vi "lab7_Avoid obstacle button2.0 - kpfinal.vi"() -> ()   [LabVIEW 2018]
uses:
  <userlib>/KNR OS 3.0 LabVIEW Toolkit/Type Definition/Resource.ctl
  <userlib>/KNR OS 3.0 LabVIEW Toolkit/Type Definition/DC Motor Port.ctl
  <userlib>/KNR OS 3.0 LabVIEW Toolkit/Type Definition/Ultrasonic Port Number.ctl
  <vilib>/myRIO/Common/Instrument Driver Framework/myRIO v1.0/UART/vis/myRIO v1.0 Close UART.vi
  <vilib>/myRIO/Common/Instrument Driver Framework/Utilities/vis/FPGA Ref Manager.vi
  <vilib>/myRIO/Common/Instrument Driver Framework/myRIO v1.0/myRIO v1.0 Reset FPGA.vi
  <vilib>/myRIO/Common/Instrument Driver Framework/myRIO v1.0/IRQ/vis/myRIO v1.0 IRQ Info FGV.vi
  <vilib>/myRIO/Common/Instrument Driver Framework/myRIO v1.0/IRQ/vis/myRIO v1.0 Timer IRQ Info FGV.vi
  <vilib>/myRIO/Common/Instrument Driver Framework/myRIO v1.0/IRQ/vis/myRIO v1.0 ISR Agent.vi
  <vilib>/myRIO/Instrument Drivers/Utilities/Utilities.lvlib
panel:
  out "Velocity R (cm/s)":dbl=3750.0
  out "Velocity L":dbl=-2062.5
  in  "stop":bool
  in  "kp":dbl=5.8 format="%#_13g"
  out "Speed R 2":dbl=4.06
  out "Speed L 2":dbl=4.06
  in  "upper limit R":dbl=15.0
  in  "upper limit L":dbl=20.0
  in  "Speed":dbl=8.0
  in  "Distance":dbl=35.0
  in  "Kp":dbl=0.3
  in  "Reverse Encoder R":bool=TRUE
  in  "Reverse Encoder L":bool=TRUE
  in  "Y":dbl=-5.0
  in  "X":dbl=190.0
  out "Pos R":dbl=170.41358455446547
  out "Pos L":dbl=162.57741982327175
  out "Actual X":dbl=165.0804505801855
  out "Actual Y":dbl=-0.734330747670838
  out "Theta":dbl=21.37996031746032 caption="Heading"
  in  "Reset Encoder R":bool
  in  "Reset Encoder L":bool
  in  "L set Us":dbl=45.0 format="%#_13g"
  in  "Mid set IR":dbl=46.0 format="%#_13g"
  in  "R set Us":dbl=25.0 format="%#_13g"
  out "Case":dbl
  out "L":dbl(slide)=299.99420158565044 scale=0.0..300.0
  out "mid":dbl(slide)=1010.0268999999998 scale=0.0..300.0
  out "R":dbl(slide)=262.09784746170044 scale=0.0..300.0
  out "L Us":dbl=299.99420158565044
  out "MID Us":dbl=1010.0268999999998
  out "R Us":dbl=262.09784746170044
  in  "?":bool
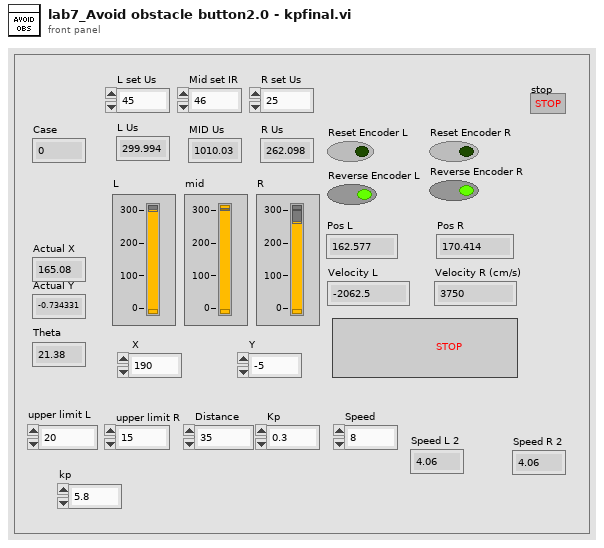
[diagram p1: front panel]
types:
  T1 = typedef "DC Motor Port.ctl" = u16
  T2 = typedef "Resource.ctl" = enum16{"KNRm_DDRC", "KNRm_DDDD", "KNRm_DDDR", "KNRm_DDDC", "KNR"}
  T3 = typedef "KNR3 Reference.ctl" = cluster{"FPGA Session":refnum<class "FPGA Interface Base.lvclass">, "Resource":T2}
  T4 = typedef "Ultrasonic Port Number.ctl" = u16
  T5 = cluster{"Dist 1(cm)":dbl, "Dist 2(cm)":dbl, "Dist 3 (cm)":dbl, "Dist 4 (cm)":dbl}
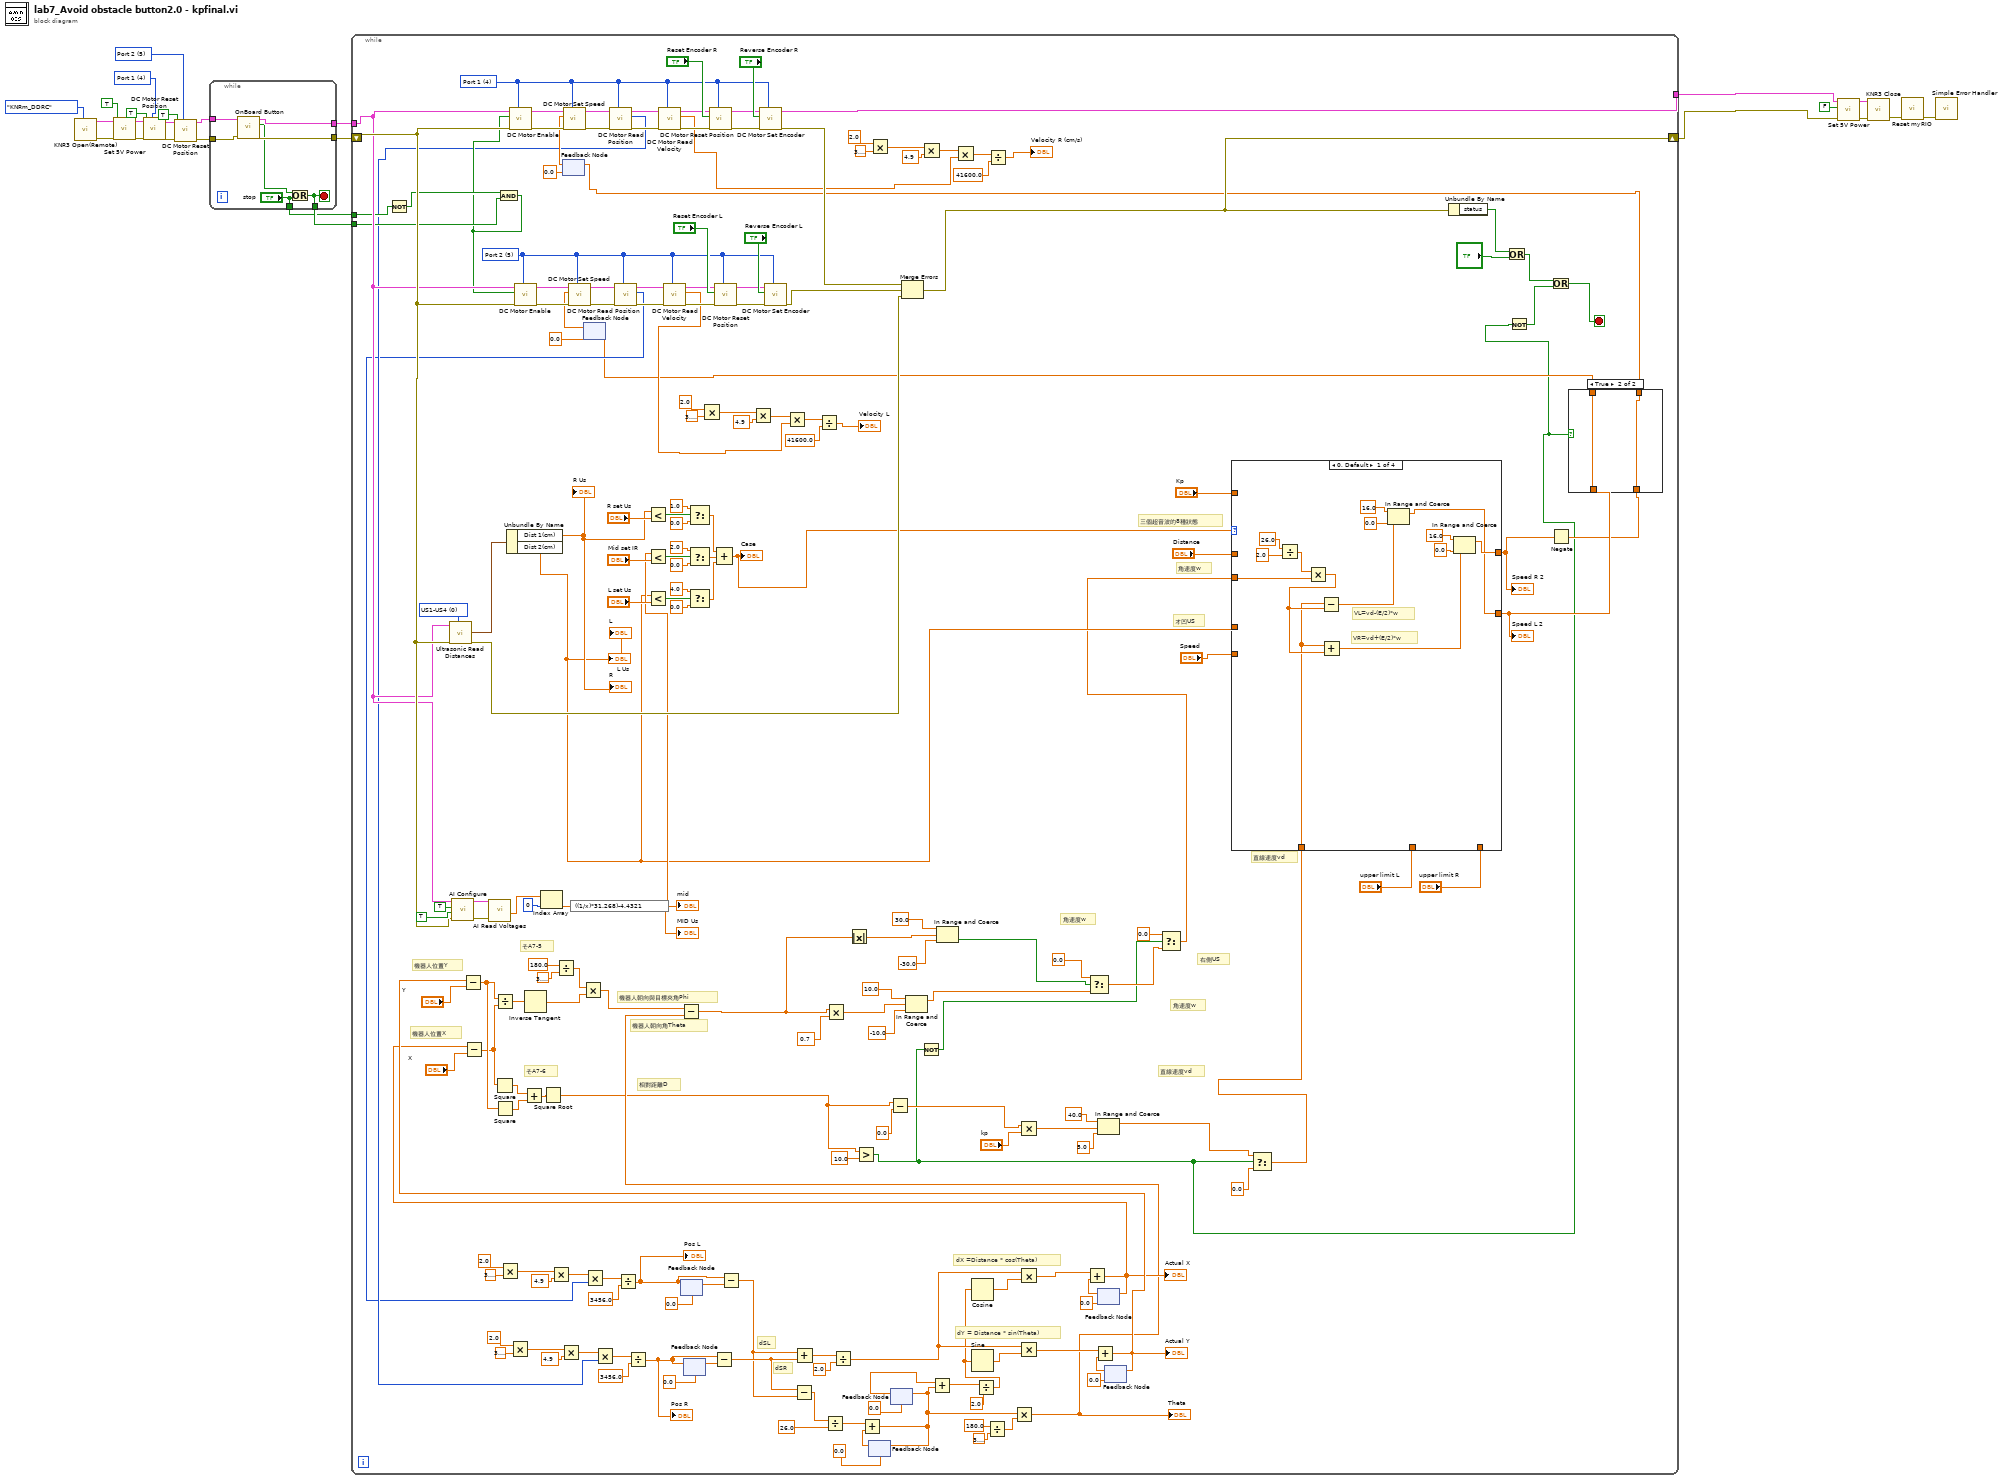
[diagram p0: block diagram]
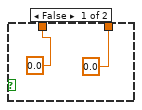
[diagram p2: hidden frame]
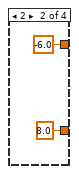
[diagram p3: hidden frame]
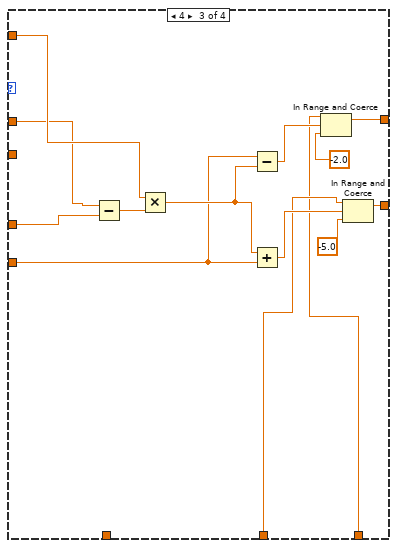
[diagram p4: hidden frame]
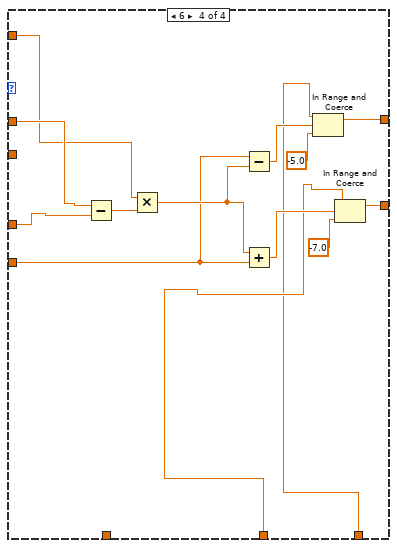
[diagram p5: hidden frame]
diagram:
  w11 = T1 5 items=["Port 1"=4, "Port 2"=5, "Port 3"=6, "Port 4"=7, "Port 5"=8, "Port 6"=9, "Port 7"=10] ("Port Number 2")
  w12 = T1 4 items=["Port 1"=4, "Port 2"=5, "Port 3"=6, "Port 4"=7, "Port 5"=8, "Port 6"=9, "Port 7"=10] ("Port Number")
  n1 = call <userlib>:"KNR3 Open(Remote).vi"("Resource"=Resource."KNRm_DDRC") -> ("error out"=w20:errorcluster, "KNR out"=w21:T3)  [unwired: 9 in]
  n2 = call <userlib>:"Set 5V Power.vi"("error in (no error)"=w20, "5V Power(T)"=TRUE ("5V Power"), "KNR in"=w21) -> ("error out"=w13:errorcluster, "KNR out"=w16:T3)  [unwired: 7 in]
  n3 = call <userlib>:"DC Motor Reset Position.vi"("Port (DS1)"=w12, "error in (no error)"=w13, "Reset(F)"=TRUE, "KNR in"=w16) -> ("error out"=w14:errorcluster, "KNR out"=w15:T3)  [unwired: 6 in]
  n4 = call <userlib>:"DC Motor Reset Position.vi"("Port (DS1)"=w11, "error in (no error)"=w14, "Reset(F)"=TRUE, "KNR in"=w15) -> ("error out"=w7:errorcluster, "KNR out"=w6:T3)  [unwired: 6 in]
  n5 = while {
    tunnel: [w32] -> w8
    tunnel: w7 -> [w31]
    tunnel: w6 -> [w30]
    tunnel: [w29] -> w5
    tunnel: [w27] -> w4
    tunnel: ["stop"] -> w3
    stop <- w27 stop-if-true
    n6 = call <userlib>:"OnBoard Button.vi"("error in (no error)"=w31, "KNR in"=w30) -> ("error out"=w32:errorcluster, "value"=w28:bool, "KNR out"=w29:T3)  [unwired: 7 in]
    n7 = Or(x=w28, y="stop") -> (x .or. y?=w27:bool)
  }
  n8 = while {
    tunnel: [w219] -> w2
    shift-right: [w205] -> w1
    shift-left: w8 -> [w168]
    tunnel: w5 -> [w91]
    tunnel: w4 -> [w90]
    tunnel: w3 -> [w89]
    stop <- w40 stop-if-true
    w204 = T4 0 items=["US1-US4"=0, "US5-US8"=2] ("Port Number")
    w208 = T1 5 items=["Port 1"=4, "Port 2"=5, "Port 3"=6, "Port 4"=7, "Port 5"=8, "Port 6"=9, "Port 7"=10] ("Port Number 2")
    w216 = T1 4 items=["Port 1"=4, "Port 2"=5, "Port 3"=6, "Port 4"=7, "Port 5"=8, "Port 6"=9, "Port 7"=10] ("Port Number")
    # "角速度w"
    # "直線速度vd"
    # "オ凹US"
    # "右側US"
    # "そΑ7-5"
    # "そΑ7-6"
    # "相對距離D"
    # "機器人朝向角Theta"
    # "機器人位置Y"
    # "機器人位置X"
    # "三個超音波的8種狀態"
    # "直線速度vd"
    # "角速度w"
    # "角速度w"
    # "機器人朝向與目標夾角Phi"
    # "dSR"
    # "dSL"
    # "dY = Distance * sin(Theta)"
    # "dX =Distance * cos(Theta)"
    n9 = Not(x=w89) -> (.not. x?=w88:bool)
    n10 = call <userlib>:"Ultrasonic Read Distances.vi"("Port (US1-US4 for KNR)"=w204, "error in (no error)"=w168, "KNR in"=w91) -> ("error out"=w187:errorcluster, "Ultrasonic output"=w203:T5)  [unwired: 6 in, 1 out]
    n11 = call <userlib>:"AI Configure.vi"("error in (no error)"=w168, "8-15 Single ended(T)"=TRUE, "0-7 Single ended(T)"=TRUE, "KNR in"=w91) -> ("error out"=w176:errorcluster, "KNR out"=w175:T3)  [unwired: 6 in]
    n12 = call <userlib>:"AI Read Voltages.vi"("error in (no error)"=w176, "KNR in"=w175) -> ("Voltages"=w171:dbl[])  [unwired: 6 in, 3 out]
    n13 = And(x=w88, y=w90) -> (x .and. y?=w87:bool)
    n14 = Multiply(x=2.0, y=3.141592653589793) -> (x*y=w163:dbl)
    n15 = Unbundle By Name(w203) -> ("Dist 1(cm)"=w112:dbl, "Dist 2(cm)"=w108:dbl)
    "R Us" <- w112
    "L Us" <- w108
    "R" <- w112
    "L" <- w108
    n16 = call <userlib>:"DC Motor Enable.vi"("Port (DS1)"=w216, "error in (no error)"=w168, "Enable Motor(F)"=w87, "KNR in"=w91) -> ("error out"=w224:errorcluster, "KNR out"=w186:T3)  [unwired: 6 in]
    n17 = Multiply(x=2.0, y=3.141592653589793) -> (x*y=w156:dbl)
    n18 = call <userlib>:"DC Motor Enable.vi"("Port (DS1)"=w208, "error in (no error)"=w168, "Enable Motor(F)"=w87, "KNR in"=w91) -> ("error out"=w215:errorcluster, "KNR out"=w177:T3)  [unwired: 6 in]
    n19 = Index Array(array=w171, index=0) -> (element=w170:dbl)
    n20 = Multiply(x=w163, y=4.9 ("wheel radius (cm)")) -> (x*y=w161:dbl)
    n21 = Divide(x=180.0, y=3.141592653589793) -> (x/y=w117:dbl)
    n22 = Multiply(x=w156, y=4.9 ("wheel radius (cm)")) -> (x*y=w154:dbl)
    n23 = feedback #1(0.0) -> (w111:dbl)
    n24 = call <userlib>:"DC Motor Set Speed.vi"("Port (DS1)"=w216, "error in (no error)"=w224, "Speed (+-100%)"=w111, "KNR in"=w186) -> ("error out"=w223:errorcluster, "KNR out"=w185:T3)  [unwired: 6 in]
    n25 = expression code="((1/x)*31.268)-4.4321"(w170) -> (w169:dbl)
    "MID Us" <- w169
    "mid" <- w169
    n26 = feedback #2(0.0 ("upper limit L")) -> (w110:dbl)
    n27 = call <userlib>:"DC Motor Set Speed.vi"("Port (DS1)"=w208, "error in (no error)"=w215, "Speed (+-100%)"=w110, "KNR in"=w177) -> ("error out"=w214:errorcluster, "KNR out"=w178:T3)  [unwired: 6 in]
    n28 = call <userlib>:"DC Motor Read Position.vi"("Port (DS1)"=w216, "error in (no error)"=w223, "KNR in"=w185) -> ("error out"=w222:errorcluster, "Position"=w67:i32, "KNR out"=w184:T3)  [unwired: 6 in]
    n29 = Multiply(x=w154, y=w67) -> (x*y=w159:dbl)
    n30 = call <userlib>:"DC Motor Read Position.vi"("Port (DS1)"=w208, "error in (no error)"=w214, "KNR in"=w178) -> ("error out"=w213:errorcluster, "Position"=w66:i32, "KNR out"=w179:T3)  [unwired: 6 in]
    n31 = Multiply(x=w161, y=w66) -> (x*y=w166:dbl)
    n32 = Divide(x=w166, y=3456.0 ("Counts per rev")) -> (x/y=w129:dbl)
    "Pos L" <- w129
    n33 = Divide(x=w159, y=3456.0 ("Counts per rev")) -> (x/y=w130:dbl)
    "Pos R" <- w130
    n34 = Less?(x=w112, y="R set Us") -> (x < y?=w199:bool)
    n35 = Less?(x=w169, y="Mid set IR") -> (x < y?=w198:bool)
    n36 = Less?(x=w108, y="L set Us") -> (x < y?=w197:bool)
    n37 = call <userlib>:"DC Motor Read Velocity.vi"("Port (DS1)"=w216, "error in (no error)"=w222, "KNR in"=w184) -> ("error out"=w221:errorcluster, "Velocity (cts/sec)"=w69:dbl, "KNR out"=w183:T3)  [unwired: 6 in]
    n38 = call <userlib>:"DC Motor Read Velocity.vi"("Port (DS1)"=w208, "error in (no error)"=w213, "KNR in"=w179) -> ("error out"=w212:errorcluster, "Velocity (cts/sec)"=w79:dbl, "KNR out"=w180:T3)  [unwired: 6 in]
    n39 = feedback #3(0.0 ("Left Wheel Distance")) -> (w144:dbl)
    n40 = feedback-in #3(w129) -> ()
    n41 = feedback #4(0.0 ("Right Wheel Distance")) -> (w143:dbl)
    n42 = feedback-in #4(w130) -> ()
    n43 = Select(t=1.0, s=w199, f=0.0) -> (s? t:f=w189:dbl)
    n44 = Select(t=2.0, s=w198, f=0.0) -> (s? t:f=w190:dbl)
    n45 = Select(t=4.0, s=w197, f=0.0) -> (s? t:f=w188:dbl)
    n46 = Multiply(x=2.0, y=3.141592653589793) -> (x*y=w82:dbl)
    n47 = call <userlib>:"DC Motor Reset Position.vi"("Port (DS1)"=w216, "error in (no error)"=w221, "Reset(F)"="Reset Encoder R", "KNR in"=w183) -> ("error out"=w220:errorcluster, "KNR out"=w182:T3)  [unwired: 6 in]
    n48 = Subtract(x=w130, y=w143) -> (x-y=w140:dbl)
    n49 = call <userlib>:"DC Motor Reset Position.vi"("Port (DS1)"=w208, "error in (no error)"=w212, "Reset(F)"="Reset Encoder L", "KNR in"=w180) -> ("error out"=w211:errorcluster, "KNR out"=w181:T3)  [unwired: 6 in]
    n50 = Compound Arithmetic op=ADD(w189, w190, w188) -> (w109:dbl)
    "Case" <- w109
    n51 = Subtract(x=w129, y=w144) -> (x-y=w139:dbl)
    n52 = Multiply(x=w82, y=4.9 ("wheel radius (cm)")) -> (x*y=w80:dbl)
    n53 = call <userlib>:"DC Motor Set Encoder.vi"("Port (DS1)"=w216, "error in (no error)"=w220, "Reverse?(F)"="Reverse Encoder R", "KNR in"=w182) -> ("error out"=w206:errorcluster, "KNR out"=w219:T3)  [unwired: 6 in]
    n54 = call <userlib>:"DC Motor Set Encoder.vi"("Port (DS1)"=w208, "error in (no error)"=w211, "Reverse?(F)"="Reverse Encoder L", "KNR in"=w181) -> ("error out"=w207:errorcluster)  [unwired: 6 in, 1 out]
    n55 = Multiply(x=w80, y=w79) -> (x*y=w85:dbl)
    n56 = Subtract(x=w140, y=w139) -> (x-y=w150:dbl)
    n57 = Add(x=w139, y=w140) -> (x+y=w148:dbl)
    n58 = Divide(x=w85, y=41600.0 ("Counts per rev")) -> (x/y=→"Velocity L":dbl)
    n59 = Divide(x=w150, y=26.0 ("Wheel Base")) -> (x/y=w137:dbl)
    n60 = Divide(x=w148, y=2.0) -> (x/y=w146:dbl)
    n61 = feedback #5(0.0) -> (w138:dbl)
    n62 = Add(x=w137, y=w138) -> (x+y=w92:dbl)
    n63 = feedback-in #5(w92) -> ()
    n64 = Multiply(x=2.0, y=3.141592653589793) -> (x*y=w73:dbl)
    n65 = feedback #6(0.0) -> (w101:dbl)
    n66 = feedback-in #6(w92) -> ()
    n67 = Merge Errors(w206, w207, w187) -> (w205:errorcluster)
    n68 = Multiply(x=w73, y=4.9 ("wheel radius (cm)")) -> (x*y=w71:dbl)
    n69 = Add(x=w92, y=w101) -> (x+y=w99:dbl)
    n70 = Multiply(x=w71, y=w69) -> (x*y=w76:dbl)
    n71 = Divide(x=w99, y=2.0) -> (x/y=w97:dbl)
    n72 = Cosine(x=w97) -> (cos(x)=w151:dbl)
    n73 = Sine(x=w97) -> (sin(x)=w100:dbl)
    n74 = Divide(x=180.0, y=3.141592653589793) -> (x/y=w147:dbl)
    n75 = Divide(x=w76, y=41600.0 ("Counts per rev")) -> (x/y=→"Velocity R (cm/s)":dbl)
    n76 = Multiply(x=w92, y=w147) -> (x*y=w113:dbl)
    "Theta" <- w113
    n77 = Multiply(x=w146, y=w151) -> (x*y=w134:dbl)
    n78 = Multiply(x=w146, y=w100) -> (x*y=w131:dbl)
    n79 = feedback #7(0.0 ("Left Wheel Distance")) -> (w135:dbl)
    n80 = Add(x=w134, y=w135) -> (x+y=w114:dbl)
    "Actual X" <- w114
    n81 = Subtract(x=w114, y="X") -> (x-y=w121:dbl)
    n82 = Square(x=w121) -> (x^2=w120:dbl)
    n83 = feedback-in #7(w114) -> ()
    n84 = feedback #8(0.0 ("Left Wheel Distance")) -> (w132:dbl)
    n85 = Add(x=w131, y=w132) -> (x+y=w115:dbl)
    "Actual Y" <- w115
    n86 = Subtract(x=w115, y="Y") -> (x-y=w122:dbl)
    n87 = Divide(x=w122, y=w121) -> (x/y=w126:dbl)
    n88 = Square(x=w122) -> (x^2=w119:dbl)
    n89 = Add(x=w120, y=w119) -> (x+y=w118:dbl)
    n90 = Inverse Tangent(1:w126) -> (0:w123:dbl)
    n91 = Square Root(x=w118) -> (sqrt(x)=w63:dbl)
    n92 = Multiply(x=w117, y=w123) -> (x*y=w116:dbl)
    n93 = Subtract(x=w116, y=w113) -> (x-y=w51:dbl)
    n94 = Multiply(x=w51, y=0.7) -> (x*y=w41:dbl)
    n95 = Absolute Value(x=w51) -> (abs(x)=w50:dbl)
    n96 = Greater?(x=w63, y=10.0) -> (0:w33:bool)
    n97 = Subtract(x=w63, y=0.0) -> (x-y=w62:dbl)
    n98 = In Range and Coerce(upper limit=10.0, x=w41, lower limit=-10.0) -> (coerced(x)=w42:dbl)  [unwired: 1 out]
    n99 = Not(x=w33) -> (.not. x?=w34:bool)
    n100 = In Range and Coerce(upper limit=30.0, x=w50, lower limit=-30.0) -> (In Range?=w46:bool)  [unwired: 1 out]
    n101 = Multiply(x=w62, y="kp") -> (x*y=w60:dbl)
    n102 = Select(t=0.0, s=w46, f=w42) -> (s? t:f=w37:dbl)
    n103 = In Range and Coerce(upper limit=40.0, x=w60, lower limit=5.0) -> (coerced(x)=w57:dbl)  [unwired: 1 out]
    n104 = feedback-in #8(w115) -> ()
    n105 = Select(t=0.0, s=w34, f=w37) -> (s? t:f=w36:dbl)
    n106 = Select(t=w57, s=w33, f=0.0) -> (s? t:f=w107:dbl)
    n107 = case shown="0, Default" w109 {
      tunnel: w108 -> [_ _ w254 w265]
      tunnel: [w231 8.0 ("upper limit") w253 w268] -> w55
      tunnel: [w232 -6.0 ("upper limit 2") w252 w267] -> w68
      tunnel: w36 -> [w234 _ _ _]
      tunnel: w107 -> [w233 _ _ _]
      tunnel: "Kp" -> [_ _ w251 w263]
      tunnel: "Distance" -> [_ _ w250 w264]
      tunnel: "Speed" -> [_ _ w249 w266]
      tunnel: "upper limit R" -> [_ _ w247 w261]
      tunnel: "upper limit L" -> [_ _ w248 w262]
      frame 0, Default {
        # "VR=vd+(E/2)*w"
        # "VL=vd-(E/2)*w"
        n108 = Divide(x=26.0, y=2.0) -> (x/y=w243:dbl)
        n109 = Multiply(x=w243, y=w234) -> (x*y=w244:dbl)
        n110 = Subtract(x=w233, y=w244) -> (x-y=w238:dbl)
        n111 = Add(x=w233, y=w244) -> (x+y=w235:dbl)
        n112 = In Range and Coerce(upper limit=16.0, x=w238, lower limit=0.0) -> (coerced(x)=w231:dbl)  [unwired: 1 out]
        n113 = In Range and Coerce(upper limit=16.0, x=w235, lower limit=0.0) -> (coerced(x)=w232:dbl)  [unwired: 1 out]
      }
      frame 2 {
      }
      frame 4 {
        n114 = Subtract(x=w250, y=w254) -> (x-y=w260:dbl)
        n115 = Multiply(x=w251, y=w260) -> (x*y=w259:dbl)
        n116 = Subtract(x=w249, y=w259) -> (x-y=w256:dbl)
        n117 = Add(x=w259, y=w249) -> (x+y=w255:dbl)
        n118 = In Range and Coerce(upper limit=w247, x=w256, lower limit=-2.0) -> (coerced(x)=w252:dbl)  [unwired: 1 out]
        n119 = In Range and Coerce(upper limit=w248, x=w255, lower limit=-5.0) -> (coerced(x)=w253:dbl)  [unwired: 1 out]
      }
      frame 6 {
        n120 = Subtract(x=w264, y=w265) -> (x-y=w274:dbl)
        n121 = Multiply(x=w263, y=w274) -> (x*y=w273:dbl)
        n122 = Subtract(x=w266, y=w273) -> (x-y=w270:dbl)
        n123 = Add(x=w273, y=w266) -> (x+y=w269:dbl)
        n124 = In Range and Coerce(upper limit=w261, x=w270, lower limit=-5.0) -> (coerced(x)=w267:dbl)  [unwired: 1 out]
        n125 = In Range and Coerce(upper limit=w262, x=w269, lower limit=-7.0) -> (coerced(x)=w268:dbl)  [unwired: 1 out]
      }
    }
    "Speed L 2" <- w55
    "Speed R 2" <- w68
    n126 = Unbundle By Name(w205) -> ("status"=w226:bool)
    n127 = Or(x=w226, y="?") -> (x .or. y?=w39:bool)
    n128 = Not(x=w33) -> (.not. x?=w38:bool)
    n129 = Or(x=w39, y=w38) -> (x .or. y?=w40:bool)
    n130 = Negate(x=w68) -> (-x=w53:dbl)
    n131 = case shown="True" w33 {
      tunnel: w55 -> [_ w230]
      tunnel: [0.0 w230] -> w54
      tunnel: w53 -> [_ w229]
      tunnel: [0.0 w229] -> w52
      frame False {
      }
      frame True {
      }
    }
    n132 = feedback-in #1(w52) -> ()
    n133 = feedback-in #2(w54) -> ()
  }
  n134 = call <userlib>:"Set 5V Power.vi"("error in (no error)"=w1, "5V Power(T)"=FALSE ("5V Power"), "KNR in"=w2) -> ("error out"=w24:errorcluster, "KNR out"=w22:T3)  [unwired: 7 in]
  n135 = call <userlib>:"KNR3 Close.vi"("error in (no error)"=w24, "KNR in"=w22) -> ("error out"=w18:errorcluster)  [unwired: 9 in]
  n136 = call <vilib>:"Reset myRIO.vi"("error in (no error)"=w18) -> ("error out"=w17:errorcluster)  [unwired: 10 in]
  n137 = call <vilib>:"Simple Error Handler.vi"("error in (no error)"=w17) -> ()  [unwired: 4 in, 5 out]
